vi "average_2_if.vi"(8 "valid2":bool, 9 "midpoint2":fxp<+,49,40>, 10 "valid1":bool, 11 "midpoint1":fxp<+,48,40>) -> (1 "valid":bool, 2 "timestamp":fxp<+,48,41>)   [LabVIEW 2018]
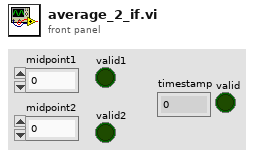
[diagram p1: front panel]
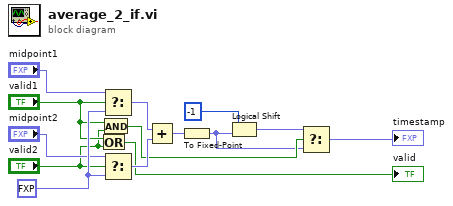
[diagram p0: block diagram]
diagram:
  w14 = fxp<+,1,1> 0.0 ("f")
  n1 = Or(x="valid1", y="valid2") -> (x .or. y?=→"valid":bool)
  n2 = And(x="valid1", y="valid2") -> (x .and. y?=w2:bool)
  n3 = Select(t="midpoint1", s="valid1", f=w14) -> (s? t:f=w12:fxp<+,48,40>)
  n4 = Select(t="midpoint2", s="valid2", f=w14) -> (s? t:f=w13:fxp<+,49,40>)
  n5 = Add(x=w12, y=w13) -> (x+y=w11:fxp<+,50,41>)
  n6 = To Fixed-Point(number=w11) -> (fixed-point=w1:fxp<+,43,41>)  [unwired: 1 in]
  n7 = Logical Shift(y=i16 -1, x=w1) -> (x << y=w9:fxp<+,43,41>)
  n8 = Select(t=w9, s=w2, f=w1) -> (s? t:f=→"timestamp":fxp<+,43,41>)
